vi "Get Measurement Times.vi"(8 "error in (no error)":errorcluster, 11 "Skyworks - 2G PVT in":refnum<class "Skyworks - PVT.lvclass">) -> (0 "error out":errorcluster, 3 "Skyworks - 2G PVT out":refnum<class "Skyworks - PVT.lvclass">)   [LabVIEW 2018, in "Skyworks PVT.lvlib" / "Skyworks - PVT.lvclass"]
uses:
  Skyworks - PVT.lvclass
  C:/Sequence Automation/Plugins/Measurement Interface.lvlibp/Measurement Interface.lvclass
  Skyworks - PVT.lvclass/Skyworks - PVT.ctl
  Plugins/Measurement Interface.lvlibp/Private Methods/Measurement Parameters/Read Measurement Parameters.vi
  Plugins/String Database.lvlibp/String Database.lvclass
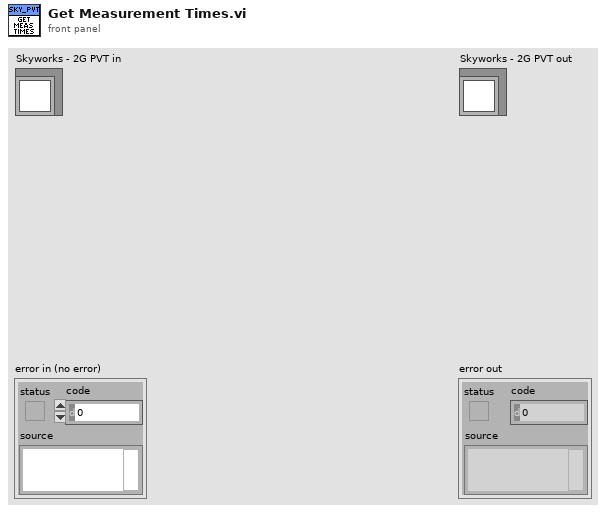
[diagram p1: front panel]
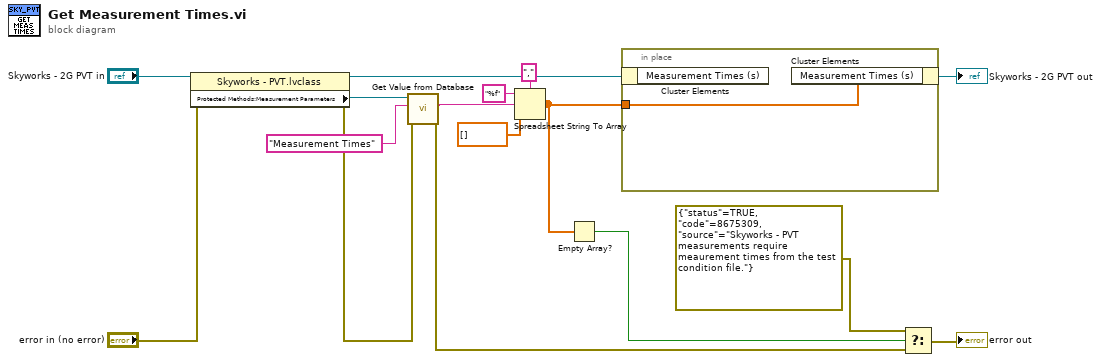
[diagram p0: block diagram]
diagram:
  n1 = property class="Skyworks - PVT.lvclass"(reference="Skyworks - 2G PVT in", error in="error in (no error)") -> (reference out=w13:refnum<class "Skyworks - PVT.lvclass">, error out=w10:errorcluster, "Protected Methods:Measurement Parameters"=w12:refnum<class "String Database.lvclass">)
  n2 = call "Get Value from Database.vi"("error in (no error)"=w10, "Entry Name"="Measurement Times", "Message in"=w12) -> ("error out"=w4:errorcluster, "Entry Value"=w9:string)  [unwired: 5 in, 2 out]
  n3 = Spreadsheet String To Array(delimiter (Tab)=",", format string="%f", spreadsheet string=w9, array type (2D Dbl)=dbl[] []) -> (array=w5:dbl[])
  n4 = Empty Array?(array=w5) -> (empty?=w3:bool)
  n5 = in-place {
    in-place-border: w5 -> [w17]
    n6 = in-place-cluster #1(w13) -> ()  [unwired: 1 out]
    n7 = in-place-cluster #1("Measurement Times (s)"=w17) -> (→"Skyworks - 2G PVT out":refnum<class "Skyworks - PVT.lvclass">)
  }
  n8 = Select(t=errorcluster {"status"=TRUE, "code"=8675309, "source"="Skyworks - PVT measurements require meaurement times from the test condition file."}, s=w3, f=w4) -> (s? t:f=→"error out":errorcluster)
